vi "RVHR - Get Current Images.vi"(6 "Local Data in":T2, 7 "UI Refs":T1, 8 "error in (no error)":errorcluster) -> (0 "error out":errorcluster, 4 "Local Data out":T2)   [LabVIEW 2024]
uses:
  Controls/RVHR - Local Data.ctl
  Controls/Test Cluster.ctl
  Controls/Excluded Information.ctl
  Controls/Language.ctl
  Controls/Device_Type.ctl
  <vilib>/Utility/miscctls.llb/LVRectTypeDef.ctl
  <vilib>/Utility/miscctls.llb/LVBoundsTypeDef.ctl
  Controls/RVHR - UI Refs.ctl
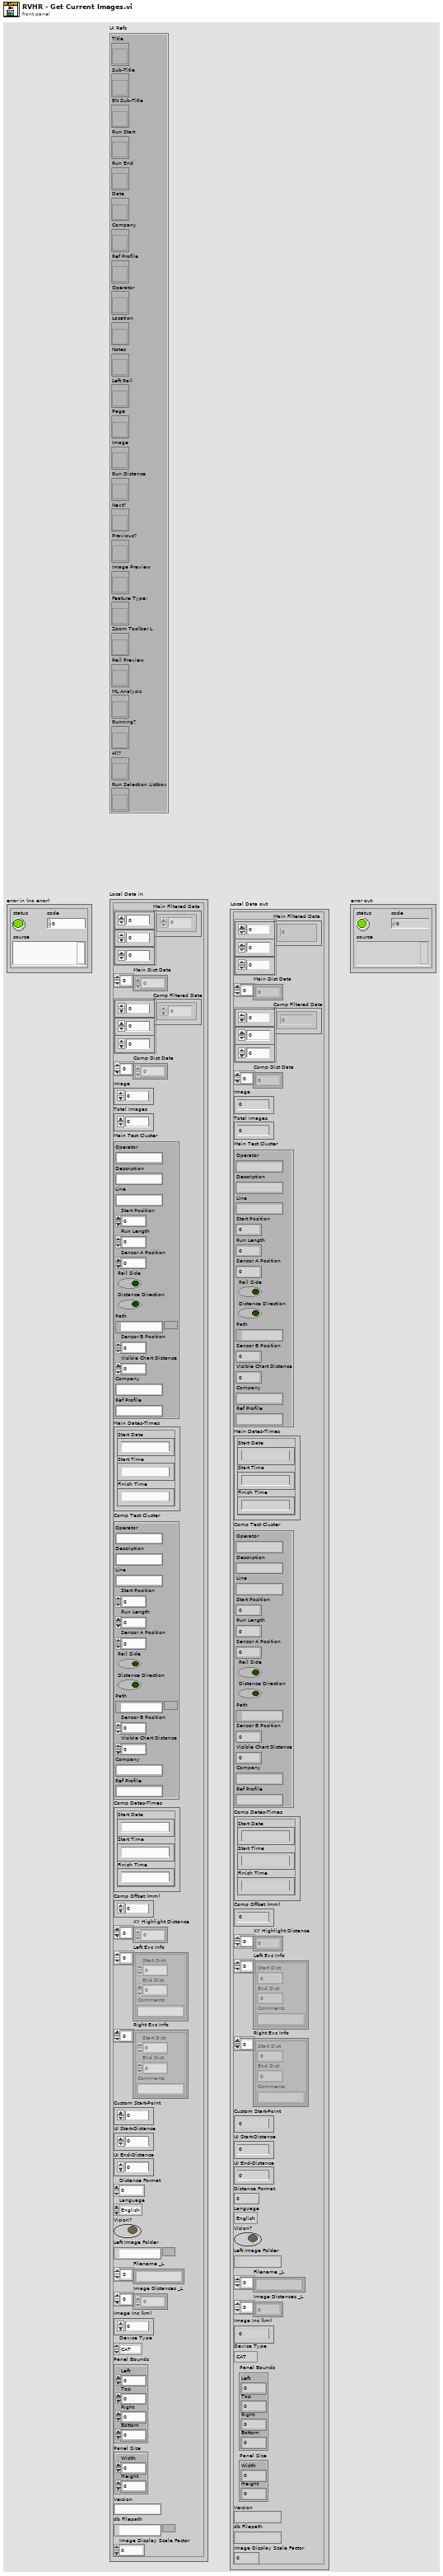
[diagram p1: front panel]
types:
  T1 = typedef "RVHR - UI Refs.ctl" = cluster{"Title":refnum<vi>, "Sub-Title":refnum<vi>, "EN Sub-Title":refnum<vi>, "Run Start":refnum<vi>, "Run End":refnum<vi>, "Date":refnum<vi>, "Company":refnum<vi>, "Ref Profile":refnum<vi>, "Operator":refnum<vi>, "Location":refnum<vi>, "Notes":refnum<vi>, "Left Rail":refnum<vi>, "Page":refnum<vi>, "Image":refnum<vi>, "Run Distance":refnum<vi>, "Next?":refnum<vi>, "Previous?":refnum<vi>, "Image Preview":refnum<vi>, "Feature Type:":refnum<vi>, "Zoom Toolbar L":refnum<vi>, "Rail Preview":refnum<vi>, "ML Analysis":refnum<vi>, "Running?":refnum<vi>, "All?":refnum<vi>, "Run Selection Listbox":refnum<vi>}
  T2 = typedef "RVHR - Local Data.ctl" = cluster{"Main Filtered Data":dbl[][][], "Main Dist Data":dbl[], "Comp Filtered Data":dbl[][][], "Comp Dist Data":dbl[], "Image":u16, "Total Images":u16, "Main Test Cluster":T3, "Main Dates-Times":cluster{"Start Date":string, "Start Time":string, "Finish Time":string}, "Comp Test Cluster":T3, "Comp Dates-Times":cluster{"Start Date":string, "Start Time":string, "Finish Time":string}, "Comp Offset (mm)":i64, "XY Highlight Distance":dbl[], "Left Exc Info":T4[], "Right Exc Info":T4[], "Custom Start-Point":dbl, "UI Start-Distance":dbl, "UI End-Distance":dbl, "Distance Format":u8, "Language":T5, "Vision?":bool, "Left Image Folder":path, "Filename _L":string[], "Image Distances _L":dbl[], "Image Inc (km)":dbl, "Device Type":T6, "Panel Bounds":T7, "Panel Size":T8, "Version":string, "db Filepath":path, "Image Display Scale Factor":dbl}
  T3 = typedef "Test Cluster.ctl" = cluster{"Operator":string, "Description":string, "Line":string, "Start Position":dbl, "Run Length":dbl, "Sensor A Position":dbl, "Rail Side":bool, "Distance Direction":bool, "Path":path, "Sensor B Position":dbl, "Visible Chart Distance":dbl, "Company":string, "Ref Profile":string}
  T4 = typedef "Excluded Information.ctl" = cluster{"Start Dist":dbl, "End Dist":dbl, "Comments":string}
  T5 = typedef "Language.ctl" = enum16{"English", "Chinese", "German"}
  T6 = typedef "Device_Type.ctl" = enum16{"CAT", "Bi-CAT", "YRCA", "RCA", "RV-HR", "TV-HR"}
  T7 = typedef "LVRectTypeDef.ctl" = cluster{"Left":i16, "Top":i16, "Right":i16, "Bottom":i16}
  T8 = typedef "LVBoundsTypeDef.ctl" = cluster{"Width":u32, "Height":u32}
  T9 = cluster{"left":i16, "top":i16, "right":i16, "bottom":i16}
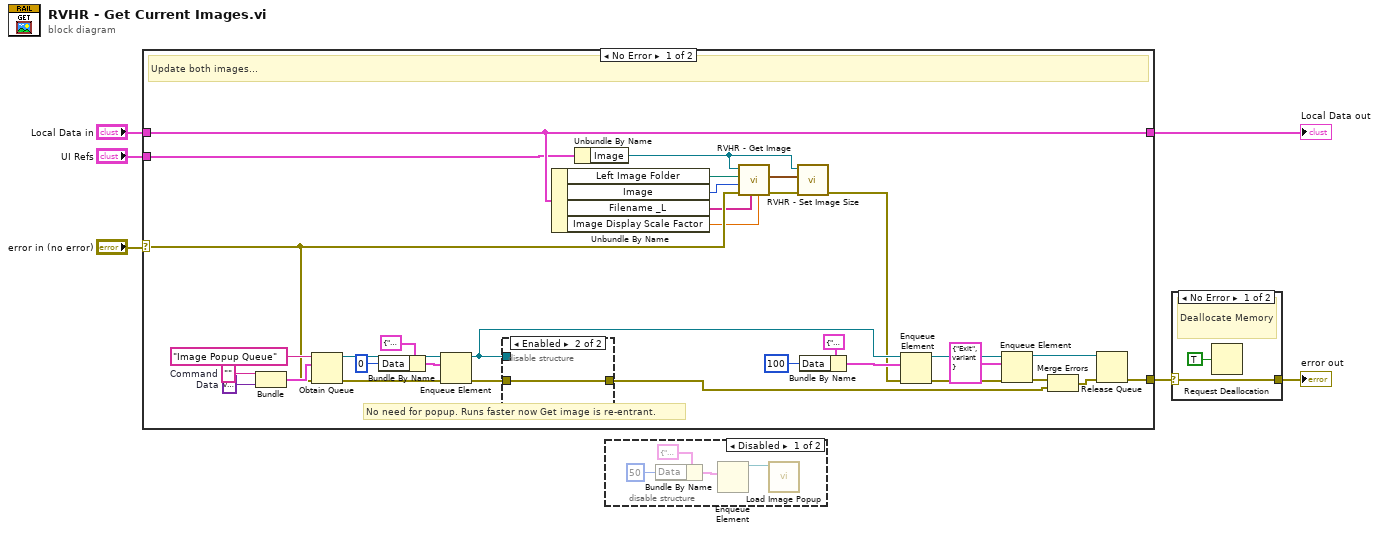
[diagram p0: block diagram]
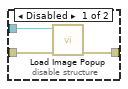
[diagram p4: hidden frame]
diagram:
  n1 = case shown="No Error" "error in (no error)" {
    selector: "error in (no error)" -> [w13 w44]
    tunnel: "UI Refs" -> [w38 _]
    tunnel: [w39 w45] -> w4
    tunnel: "Local Data in" -> [w39 w45]
    tunnel: [w30 w44] -> w2
    frame No Error {
      w27 = variant  # Data
      w28 = ""  # Command
      # "No need for popup. Runs faster now Get image is re-entrant."
      # "Update both images..."
      n2 = Bundle("Command"=w28, "Data"=w27) -> (w29:cluster{"Command":string, "Data":variant})  [unwired: 1 in]
      n3 = Obtain Queue(name (unnamed)="Image Popup Queue", element data type=w29, error in (no error)=w13) -> (queue out=w24:refnum<queue>, error out=w25:errorcluster)  [unwired: 2 in, 1 out]
      n4 = Bundle By Name(cluster=cluster{"Command":string, "Data":variant} {"Command"="Update Progress", "Data"=variant} ("output cluster"), "Data"=u8 0 ("Progress")) -> (w34:cluster{"Command":string, "Data":variant})
      n5 = Enqueue Element(queue=w24, element=w34, error in (no error)=w25) -> (queue out=w17:refnum<queue>, error out=w31:errorcluster)  [unwired: 1 in, 1 out]
      n6 = disable-structure shown="Enabled" {
        disable-tunnel: w31 -> [w42 w43]
        disable-tunnel: w17 -> [w41 _]
        disable-tunnel: [w40 w43] -> w16
        frame Disabled {
          n7 = call "Load Image Popup.vi"("error in"=w42, "queue in"=w41) -> ("error out"=w40:errorcluster)  [unwired: 8 in, 1 out]
        }
        frame Enabled {
        }
      }
      n8 = Unbundle By Name(w39) -> ("Left Image Folder"=w11:path, "Image"=w7:u16, "Filename _L"=w12:string[], "Image Display Scale Factor"=w8:dbl)
      n9 = Unbundle By Name(w38) -> ("Image"=w9:refnum<vi>)
      n10 = call "RVHR - Get Image.vi"("Scale Factor"=w8, "Filename _L"=w12, "error in (no error)"=w13, "Image #"=w7, "Left Image Folder"=w11, "Image"=w9) -> ("error out"=w14:errorcluster, "Rectangle"=w10:T9)  [unwired: 4 in]
      n11 = call "RVHR - Set Image Size.vi"("error in (no error)"=w14, "Rectangle"=w10, "Image_L"=w9) -> ("error out"=w15:errorcluster)  [unwired: 8 in]
      n12 = Bundle By Name(cluster=cluster{"Command":string, "Data":variant} {"Command"="Update Progress", "Data"=variant} ("output cluster"), "Data"=u8 100 ("Progress")) -> (w37:cluster{"Command":string, "Data":variant})
      n13 = Enqueue Element(queue=w17, element=w37, error in (no error)=w15) -> (queue out=w22:refnum<queue>, error out=w21:errorcluster)  [unwired: 1 in, 1 out]
      n14 = Enqueue Element(queue=w22, element=cluster{"Command":string, "Data":variant} {"Command"="Exit", "Data"=variant} ("output cluster"), error in (no error)=w21) -> (queue out=w20:refnum<queue>, error out=w19:errorcluster)  [unwired: 1 in, 1 out]
      n15 = Merge Errors(w19, w16) -> (w18:errorcluster)
      n16 = Release Queue(queue=w20, error in (no error)=w18) -> (error out=w30:errorcluster)  [unwired: 1 in, 2 out]
    }
    frame Error {
    }
  }
  "Local Data out" <- w4
  n17 = disable-structure shown="Disabled" {
    frame Disabled {
      n18 = Bundle By Name(cluster=cluster{"Command":string, "Data":variant} {"Command"="Update Progress", "Data"=variant} ("output cluster"), "Data"=u8 50 ("Progress")) -> (w49:cluster{"Command":string, "Data":variant})
      n19 = Enqueue Element(element=w49) -> (queue out=w48:refnum<queue>)  [unwired: 3 in, 2 out]
      n20 = call "Load Image Popup.vi"("queue in"=w48) -> ()  [unwired: 9 in, 2 out]
    }
    frame Enabled {
    }
  }
  n21 = case shown="No Error" w2 {
    selector: w2 -> [w50 w52]
    tunnel: [w50 w52] -> w1
    frame No Error {
      # "Deallocate Memory"
      n22 = Request Deallocation(TRUE ("flag")) -> ()
    }
    frame Error {
    }
  }
  "error out" <- w1
